vi "SetConfig.vi"(6 "ID":string, 8 "error in (no error)":errorcluster, 9 "Port":u16, 10 "Address":string, 11 "ClientBase in":refnum<class "TCP.lvclass">) -> (0 "error out":errorcluster, 3 "ClientBase out":refnum<class "TCP.lvclass">)   [LabVIEW 2020, in "TCP.lvlib" / "TCP.lvclass"]
uses:
  TCP.lvclass
  TCP.lvclass/TCP.ctl
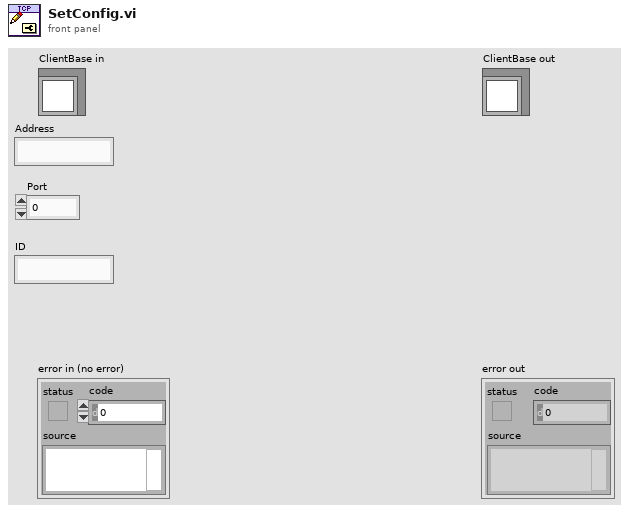
[diagram p1: front panel]
types:
  T1 = typedef "ConnectionProperties.ctl" = cluster{"Address":string, "Port":u16, "ID":string, "Connection ID":refnum<k5>, "Connected":bool, "Abort":bool}
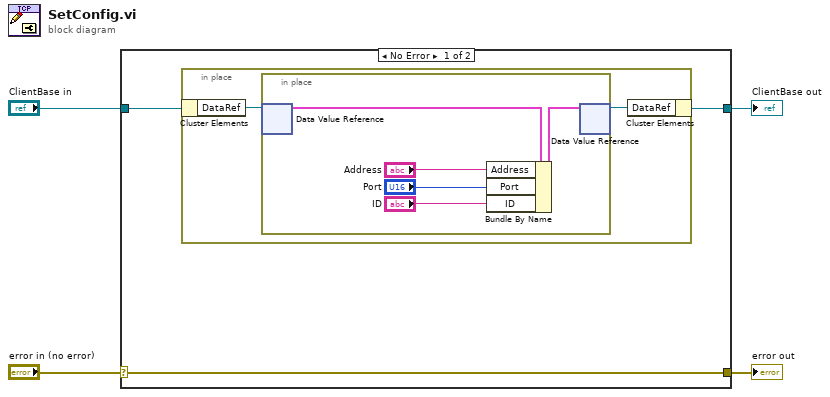
[diagram p0: block diagram]
diagram:
  n1 = case shown="No Error" "error in (no error)" {
    selector: "error in (no error)" -> [w7 w16]
    tunnel: [w7 w16] -> w3
    tunnel: [w5 w15] -> w1
    tunnel: "ClientBase in" -> [w6 w15]
    frame No Error {
      n2 = in-place {
        n3 = in-place-cluster #1(w6) -> ("DataRef"=w9:refnum<data-value>)
        n4 = in-place {
          n5 = in-place-dvr #2(w9) -> (w14:T1)  [unwired: 1 out]
          n6 = Bundle By Name(cluster=w14, "Address"="Address", "Port"="Port", "ID"="ID") -> (w13:T1)
          n7 = in-place-dvr #2(w13) -> (w8:refnum<data-value>)  [unwired: 1 out]
        }
        n8 = in-place-cluster #1("DataRef"=w8) -> (w5:refnum<class "TCP.lvclass">)
      }
    }
    frame Error {
    }
  }
  "error out" <- w3
  "ClientBase out" <- w1
